vi "listDevices.vi"(8 "error in (no error)":errorcluster, 10 "Listbox Reference":refnum<vi>, 11 "DeviceFactory in":refnum<class "DeviceFactory.lvclass">) -> (0 "error out":errorcluster, 3 "DeviceFactory out":refnum<class "DeviceFactory.lvclass">)   [LabVIEW 2020, in "DeviceFactory.lvclass"]
uses:
  DeviceFactory.lvclass
  DeviceFactory.lvclass/DeviceFactory.ctl
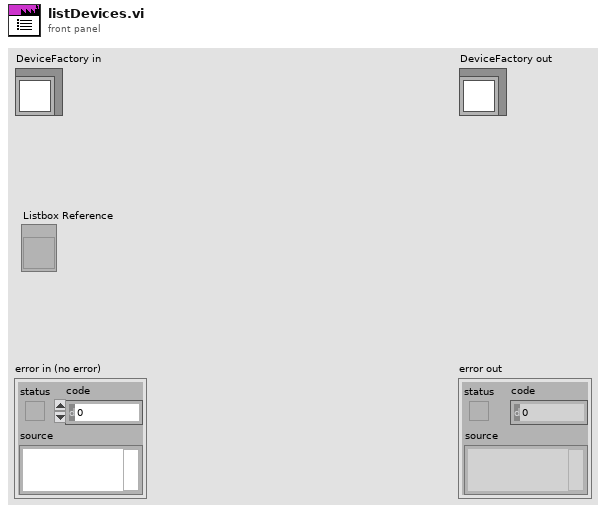
[diagram p1: front panel]
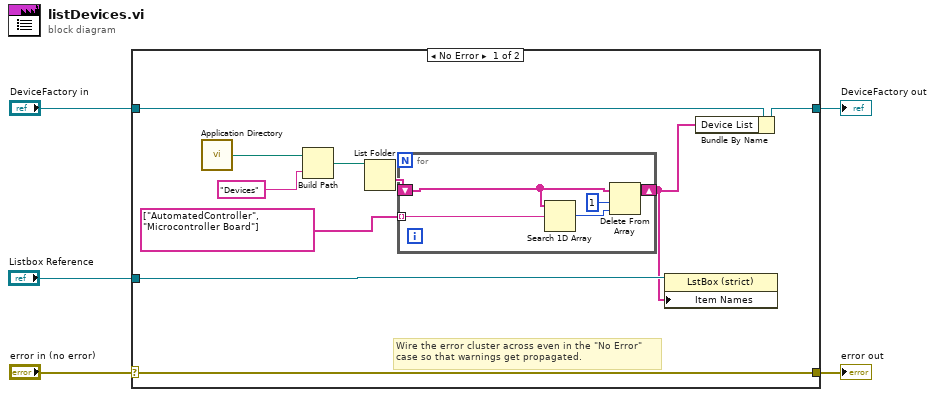
[diagram p0: block diagram]
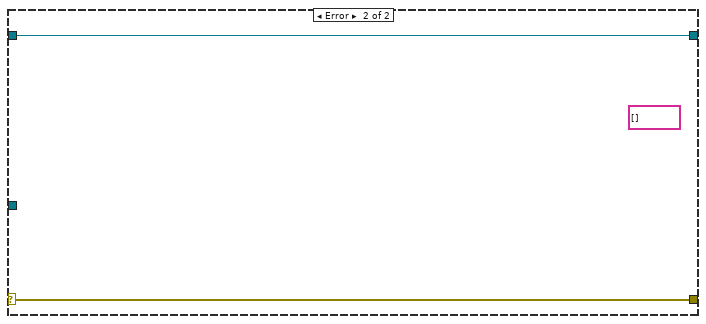
[diagram p2: hidden frame]
diagram:
  n1 = case shown="No Error" "error in (no error)" {
    selector: "error in (no error)" -> [w14 w22]
    tunnel: [w14 w22] -> w4
    tunnel: [w9 w21] -> w2
    tunnel: "DeviceFactory in" -> [w15 w21]
    tunnel: "Listbox Reference" -> [w8 _]
    frame No Error {
      # "Wire the error cluster across even in the \"No Error\"\ncase so that warnings get propagated."
      n2 = call <vilib>:"Application Directory.vi"() -> ("Application Directory"=w13:path)
      n3 = Build Path(base path=w13, name or relative path="Devices") -> (appended path=w11:path)
      n4 = List Folder(path=w11) -> (folder names=w10:string[])  [unwired: 3 in, 3 out]
      n5 = for {
        shift-right: [w17] -> w7
        shift-left: w10 -> [w18]
        tunnel: string[] ["AutomatedController", "Microcontroller Board"] ("element") -> [w16] mode=indexing
        n6 = Search 1D Array(1D array=w18, element=w16) -> (index of element=w20:i32)  [unwired: 1 in]
        n7 = Delete From Array(array=w18, length=1 ("index"), index=w20) -> (array with subset deleted=w17:string[])  [unwired: 1 out]
      }
      n8 = property class="LstBox (strict)"(reference=w8, "Item Names"=w7) -> ()  [unwired: 1 in, 2 out]
      n9 = Bundle By Name(cluster=w15, "Device List"=w7) -> (w9:refnum<class "DeviceFactory.lvclass">)
    }
    frame Error {
      (unwired) string[] [] ("folder names")
    }
  }
  "error out" <- w4
  "DeviceFactory out" <- w2
